vi "Resistance-Read.vi"(1 "Resistor":i32=10000, 2 "Input voltage":dbl) -> (0 "Resistance":dbl)   [LabVIEW 2020]
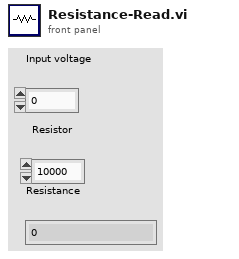
[diagram p1: front panel]
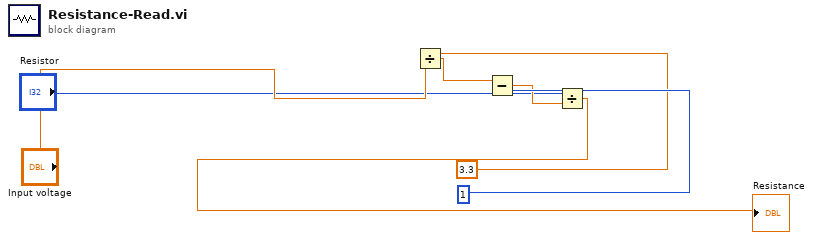
[diagram p0: block diagram]
diagram:
  n1 = Divide(x=3.3, y="Input voltage") -> (x/y=w4:dbl)
  n2 = Subtract(x=w4, y=1) -> (x-y=w5:dbl)
  n3 = Divide(x="Resistor", y=w5) -> (x/y=→"Resistance":dbl)
